vi "Read.vi"(8 "error in (no error)":errorcluster, 11 "Enum Array in":refnum<class "Enum Array.lvclass">) -> (0 "error out":errorcluster, 1 "Enum Alias Array":string[](array[string]), 2 "Enum Index Array":u32[](array[numeric]), 3 "Enum Array out":refnum<class "Enum Array.lvclass">)   [LabVIEW 2020, in "Data.lvlib" / "Enum Array.lvclass"]
doc: "Read Enum Array."
uses:
  Enum Array.lvclass
  Enum Array.lvclass/Enum Array.ctl
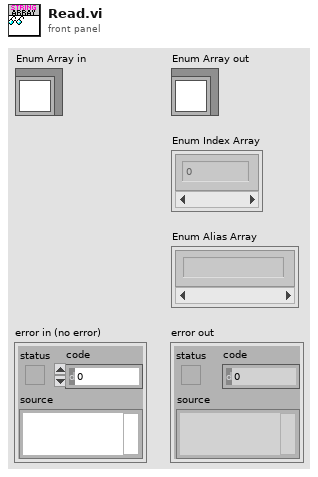
[diagram p1: front panel]
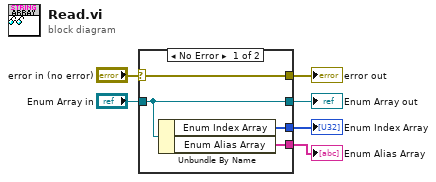
[diagram p0: block diagram]
diagram:
  n1 = case shown="No Error" "error in (no error)" {
    selector: "error in (no error)" -> [w10 w11]
    tunnel: [w10 w11] -> w5
    tunnel: [w9 w12] -> w3
    tunnel: "Enum Array in" -> [w9 w12]
    tunnel: [w8 _] -> w2
    tunnel: [w7 _] -> w1
    frame No Error {
      n2 = Unbundle By Name(w9) -> ("Enum Index Array"=w8:u32[], "Enum Alias Array"=w7:string[])
    }
    frame Error {
    }
  }
  "error out" <- w5
  "Enum Array out" <- w3
  "Enum Alias Array" <- w1
  "Enum Index Array" <- w2
